vi "Position_to_angle.vi"(8 "Set position [°]":dbl format="%#_13g", 11 "Current position [°]":dbl format="%#_13g") -> (3 "Rotation angle [°]":dbl format="%#_13g")   [LabVIEW 2018]
doc: "This VI enables to convert the set position to the rotation angle and the direction.\n\nInputs:\n(1) Set position [°] - the set position.\n(2) Current position [°] - the current position of the filter.\n\nOutput:\n(1) Rotation angle [°] - the calculated rotation angle."
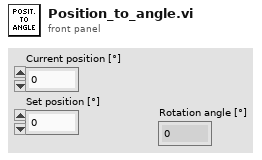
[diagram p1: front panel]
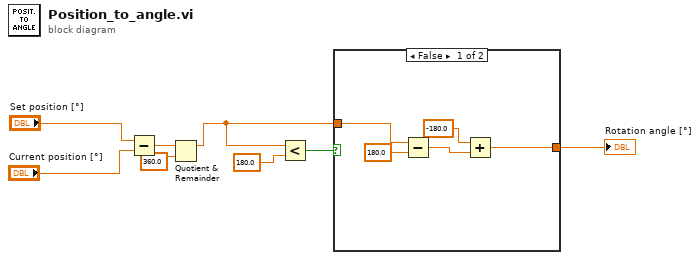
[diagram p0: block diagram]
diagram:
  n1 = Subtract(x="Set position [°]", y="Current position [°]") -> (x-y=w3:dbl)
  n2 = Quotient & Remainder(x=w3, y=360.0) -> (x-y*floor(x/y)=w1:dbl)  [unwired: 1 out]
  n3 = Less?(x=w1, y=180.0) -> (x < y?=w7:bool)
  n4 = case shown="False" w7 {
    tunnel: [w13 w14] -> w6
    tunnel: w1 -> [w9 w14]
    frame False {
      n5 = Subtract(x=w9, y=180.0) -> (x-y=w12:dbl)
      n6 = Add(x=-180.0, y=w12) -> (x+y=w13:dbl)
    }
    frame True {
    }
  }
  "Rotation angle [°]" <- w6
